vi "Benchmark Custom 1.vi"(7 "Reinit":bool, 8 "error in (no error)":errorcluster, 9 "X0":i64, 10 "X1":i64, 11 "CIFCorePlugin in":refnum<class "CIFCorePlugin.lvclass">) -> (0 "error out":errorcluster, 3 "CIFCorePlugin out":refnum<class "CIFCorePlugin.lvclass">)   [LabVIEW 2021, in "CIFCorePlugin.lvclass"]
doc: "Load a new data value into the statistics class. The new value will be calculated by subracting the X0 value from the X1 value. This VI is useful for benchmarking where a timestamp is taken before and after a function. The results of this benchmark will automatically be reported through the plugin statistics."
uses:
  CIFCorePlugin.lvclass
  CIFCorePlugin.lvclass/CIFCorePlugin.ctl
  <vilib>/CIF Foundation/CIF Utilities/Statistics/I64/Stats_I64_CIF_U.lvclass
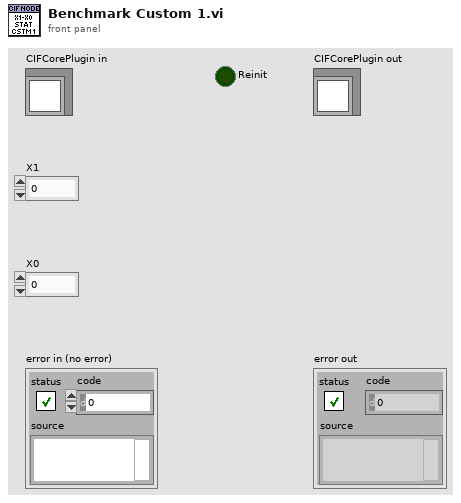
[diagram p1: front panel]
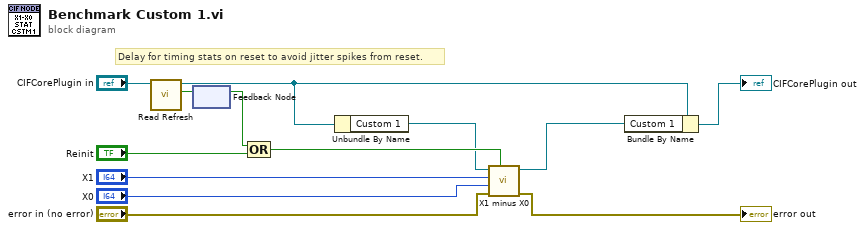
[diagram p0: block diagram]
diagram:
  # "Delay for timing stats on reset to avoid jitter spikes from reset."
  n1 = call "Read Refresh.vi"("CIFCorePlugin in"="CIFCorePlugin in") -> ("Refresh"=w2:bool, "CIFCorePlugin out"=w5:refnum<class "CIFCorePlugin.lvclass">)  [unwired: 8 in, 1 out]
  n2 = feedback-in #1(w2) -> ()
  n3 = feedback #1() -> (w1:bool)  [unwired: 1 in]
  n4 = Compound Arithmetic op=OR(w1, "Reinit") -> (w6:bool)
  n5 = Unbundle By Name(w5) -> ("Custom 1"=w4:refnum<class "Stats_I64_CIF_U.lvclass">)
  n6 = call <vilib>:"X1 minus X0.vi"("Reinit"=w6, "error in (no error)"="error in (no error)", "X0"="X0", "X1"="X1", "Stats_I64_CIF_U in"=w4) -> ("error out"=→"error out":errorcluster, "Stats_I64_CIF_U out"=w3:refnum<class "Stats_I64_CIF_U.lvclass">)  [unwired: 5 in]
  n7 = Bundle By Name(cluster=w5, "Custom 1"=w3) -> (→"CIFCorePlugin out":refnum<class "CIFCorePlugin.lvclass">)
